vi "Updater Convert All TDMS Files 5.0 to 5.1.vi"(5 "Current Version":string, 6 "Connection Refnum In":T1, 7 "Previous Version":string, 8 "error in (no error)":errorcluster, 11 "Folder Path":path) -> (0 "error out":errorcluster, 4 "Connection Refnum Out":T1)   [LabVIEW 2011]
uses:
  Summitek EXT/ODBC/SQL Controls/Connection Refnum.ctl
panel:
  in  "Continue":bool
  out "Estimated Time to Completion (min)":dbl format="%.2g"
  out "Avg Time Per File (sec)":dbl format="%.2g"
  out "Conversion Progress":u8(slide) max=21 scale=0.0..100.0
  out "Errors":string
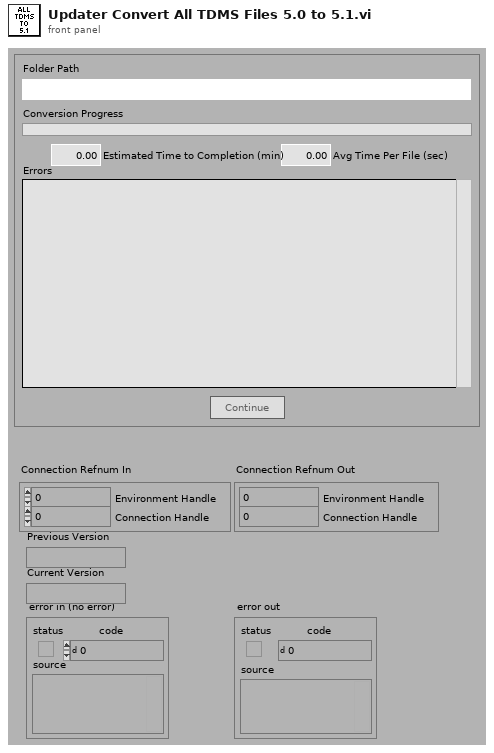
[diagram p1: front panel]
types:
  T1 = typedef "Connection Refnum.ctl" = cluster{"Environment Handle":i32, "Connection Handle":i32}
  T2 = cluster{"left":i16, "top":i16, "right":i16, "bottom":i16}
  T3 = enum8{"Enabled", "Disabled", "Disabled and Grayed Out"}
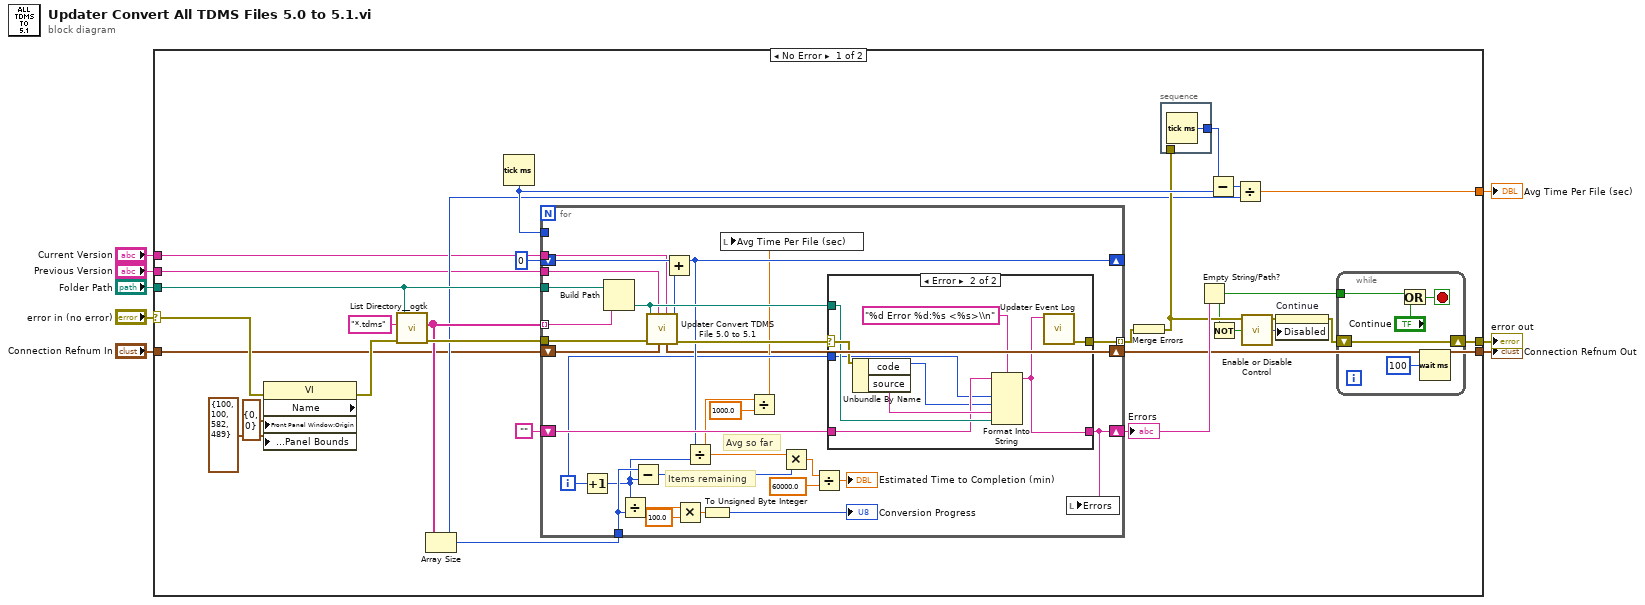
[diagram p0: block diagram]
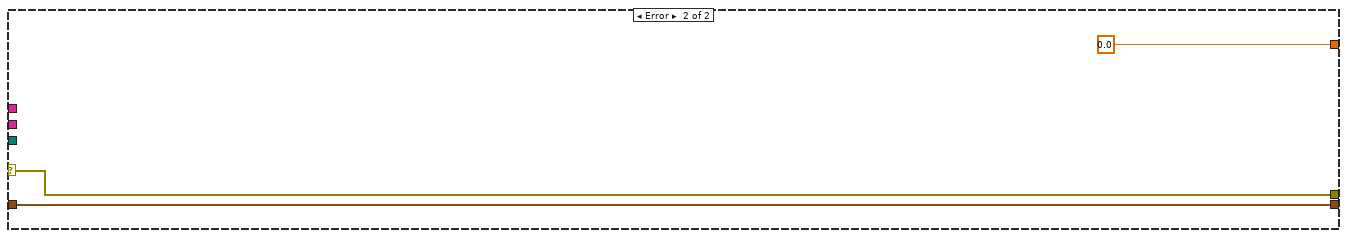
[diagram p3: hidden frame]
diagram:
  n1 = case shown="No Error" "error in (no error)" {
    selector: "error in (no error)" -> [w13 w83]
    tunnel: [w22 w83] -> w5
    tunnel: [w14 0.0] -> w8
    tunnel: "Folder Path" -> [w29 _]
    tunnel: "Current Version" -> [w12 _]
    tunnel: "Previous Version" -> [w11 _]
    tunnel: "Connection Refnum In" -> [w10 w82]
    tunnel: [w9 w82] -> w1
    frame No Error {
      n2 = property class="VI" props=["Name", "Front Panel Window:Origin", "Front Panel Window:Panel Bounds"](error in=w13, "Front Panel Window:Origin"=cluster{"Horizontal":i16, "Vertical":i16} {"Horizontal"=0, "Vertical"=0}, "Front Panel Window:Panel Bounds"=T2 {"left"=100, "top"=100, "right"=582, "bottom"=489}) -> (error out=w23:errorcluster)  [unwired: 1 in, 2 out]
      n3 = call "List Directory__ogtk.vi"("error in (no error)"=w23, "pattern"="*.tdms", "directory path"=w29) -> ("error out"=w34:errorcluster, "file names"=w32:string[])  [unwired: 3 out]
      n4 = Array Size(array=w32) -> (size(s)=w15:i32)
      n5 = Tick Count (ms)() -> (millisecond timer value=w26:u32)
      n6 = for {
        tunnel: w29 -> [w70]
        tunnel: w32 -> [w69] mode=indexing
        tunnel: w34 -> [w68]
        tunnel: [w62] -> w33 mode=indexing
        tunnel: w15 -> [w57]
        shift-right: [w49] -> w21
        shift-left: "" -> [w60]
        shift-right: [w52] -> _
        shift-left: u32 0 ("y") -> [w59]
        tunnel: w26 -> [_]
        tunnel: w12 -> [w45]
        tunnel: w11 -> [w44]
        shift-right: [w42] -> w9
        shift-left: w10 -> [w43]
        i -> [w50]
        # "Avg so far"
        # "Items remaining"
        n7 = Increment(x=w50) -> (x+1=w51:i32)
        n8 = Build Path(base path=w70, name or relative path=w69) -> (appended path=w61:path)
        n9 = Divide(x=w51, y=w57) -> (x/y=w67:dbl)
        n10 = Subtract(x=w57, y=w51) -> (x-y=w56:i32)
        n11 = call "Updater Convert TDMS File 5.0 to 5.1.vi"("Current Version"=w45, "Connection Refnum In"=w43, "Previous Version"=w44, "error in (no error)"=w68, "TDMS Path"=w61) -> ("error out"=w63:errorcluster, "Conversion Time (ms)"=w58:u32, "Connection Refnum Out"=w42:T1)  [unwired: 1 in, 3 out]
        n12 = Add(x=w59, y=w58) -> (x+y=w52:u32)
        n13 = Multiply(x=w67, y=100.0) -> (x*y=w65:dbl)
        n14 = Divide(x=w52, y=w51) -> (x/y=w47:dbl)
        n15 = To Unsigned Byte Integer(number=w65) -> (unsigned 8bit integer=→"Conversion Progress":u8)
        n16 = Divide(x=w47, y=1000.0) -> (x/y=w46:dbl)
        n17 = local write "Avg Time Per File (sec)"(w46) -> ()
        n18 = Multiply(x=w47, y=w56) -> (x*y=w55:dbl)
        n19 = Divide(x=w55, y=60000.0) -> (x/y=→"Estimated Time to Completion (min)":dbl)
        n20 = case shown="Error" w63 {
          selector: w63 -> [w72 w81]
          tunnel: [w72 w74] -> w62
          tunnel: w61 -> [_ w79]
          tunnel: w60 -> [w71 w78]
          tunnel: [w71 w73] -> w49
          tunnel: w50 -> [_ w75]
          frame No Error {
          }
          frame Error {
            n21 = Unbundle By Name(w81) -> ("code"=w76:i32, "source"=w80:string)
            n22 = Format Into String(format string="%d Error %d:%s <%s>\\n" ("pattern"), initial string=w78, w75, w76, w80, w79) -> (resulting string=w73:string)  [unwired: 1 in, 1 out]
            n23 = call "Updater Event Log.vi"("Log Entry"=w73) -> ("error out"=w74:errorcluster)  [unwired: 1 in, 9 out]
          }
        }
        n24 = local write "Errors"(w49) -> ()
      }
      "Errors" <- w21
      n25 = Merge Errors(w33) -> (w20:errorcluster)
      n26 = stacked-sequence {
        tunnel: w20 -> [_]
        tunnel: [w41] -> w31
        frame #0 {
          n27 = Tick Count (ms)() -> (millisecond timer value=w41:u32)
        }
      }
      n28 = Empty String/Path?(string/path=w21) -> (empty?=w17:bool)
      n29 = Subtract(x=w31, y=w26) -> (x-y=w30:u32)
      n30 = Not(x=w17) -> (.not. x?=w16:bool)
      n31 = Divide(x=w30, y=w15) -> (x/y=w14:dbl)
      n32 = call "Enable or Disable Control.vi"("Enable? (T)"=w16) -> ("Enable\\Disable"=w18:T3)
      n33 = property on="Continue" class="Bool"(error in=w20, "Disabled"=w18) -> (error out=w19:errorcluster)  [unwired: 1 in, 1 out]
      n34 = while {
        shift-right: [w40] -> w22
        shift-left: w19 -> [w40]
        tunnel: w17 -> [w38]
        stop <- w36 stop-if-true
        n35 = Or(x=w38, y="Continue") -> (x .or. y?=w36:bool)
        n36 = Wait (ms)(milliseconds to wait=u32 100) -> ()  [unwired: 1 out]
      }
    }
    frame Error {
    }
  }
  "error out" <- w5
  "Avg Time Per File (sec)" <- w8
  "Connection Refnum Out" <- w1
